vi "Poll DMA.vi"(8 "error in":errorcluster, 10 "Injection.Results":T13 {"Measurements"."Shots"."Results"."Off-Stage Min Volt" format="%#.6g"; "Measurements"."Shots"."Results"."Off-Stage Avg Volt" format="%#.6g"; "Measurements"."Shots"."Results"."Off-Stage Max Volt" format="%#.6g"; "Measurements"."Shots"."Results"."Total Stage Time (us)" format="%#.6g"; "Measurements"."Shots"."Results"."Off-Stage Avg Current" format="%#.6g"; "Measurements"."Shots"."Results"."Total Voltage Pulses" format="%#.6g"; "Measurements"."Shots"."Results"."Off-Stage Min Current" format="%#.6g"; "Measurements"."Shots"."Results"."Off-Stage Max Current" format="%#.6g"}, 11 "Parameters":T1) -> (0 "error out":errorcluster, 1 "Elements Remaining":u32, 3 "Parameters":T1)   [LabVIEW 2019, in "Fuel Injector Analysis Addon Engine.lvlib"]
uses:
  Fuel Injector Analysis Addon Engine.lvlib
  Types/Injector Event Data Cluster.ctl
  Types/Shot Information Control.ctl
  Types/Stage.Measurements.ctl
  Types/Async Parameters.ctl
  Addon Shared/Types/Shot.Parameters.ctl
  Addon Shared/Types/Stage.Parameters.ctl
  Addon Shared/Types/Stage.PullIn.Types.ctl
  Addon Shared/Types/Stage.Transition.Types.ctl
  Addon Shared/Types/Analysis.Channels.Select.ctl
  Addon Shared/Types/Injector info.ctl
  Types/Injector.State.ctl
  <vilib>/NI/NIVS Inline Async API/_Data Access Engine/Data Access Engine/Types/Write.DVR.ctl
  <vilib>/NI/NIVS Inline Async API/_Data Access Engine/Access Type Classes/Write/Write.lvclass
  <vilib>/NI/NIVS Inline Async API/_Data Access Engine/Data Access Engine/Types/Read.DVR.ctl
  <vilib>/NI/NIVS Inline Async API/_Data Access Engine/Access Type Classes/Read/Read.lvclass
  Addon Shared/Types/Compiled.Group.WaveformRefs.ctl
  <vilib>/NI VeriStand/Custom Device API/Waveform Data Reference.ctl
  <vilib>/NI VeriStand/Custom Device Waveform API/Single Waveform Write (DBL)/Single Waveform Write (DBL).lvclass
  C:/Program Files (x86)/National Instruments/LabVIEW 2019/vi.lib/NI VeriStand/Custom Device Waveform API/Waveform Session.lvclass
  <vilib>/NI/NIVS Inline Async API/_Data Access Engine/Access Type Classes/Read/Read.lvclass/Read.ctl
  <vilib>/NI VeriStand/Custom Device Waveform API/Waveform Session.lvclass/Waveform Session.ctl
  <vilib>/NI VeriStand/Custom Device Waveform API/Single Waveform Write (DBL)/Single Waveform Write (DBL).lvclass/Single Waveform Write (DBL).ctl
  <vilib>/NI VeriStand/Custom Device Waveform API/Internal Comm Classes/WPL Comm/WPL Comm (1D DBL)/WPL Comm (1D DBL).lvclass/WPL Comm (1D DBL).ctl
  <vilib>/NI VeriStand/Custom Device Waveform API/Internal Comm Classes/WPL Comm/WPL Comm.lvclass/WPL Comm.ctl
  <vilib>/NI/NIVS Inline Async API/_Data Access Engine/Access Type Classes/Write/Write.lvclass/Write.ctl
  Waveform Write.vi
  Stages.GetValues.vi
  Pack Data and Write to Inline.vi
  Build Event from Shots.vi
  Parse Injection Data.vi
  <vilib>/NI VeriStand/Custom Device Waveform API/NI VeriStand - Write Waveform(s).vi
  <vilib>/NI VeriStand/Custom Device Waveform API/Single Waveform Write (DBL)/NI VeriStand - Write Single Waveform (DBL).vi
  <vilib>/NI/NIVS Inline Async API/_Data Access Engine/Data Access Engine/Methods/Data.Processes.Execute.vi
  <vilib>/NI/NIVS Inline Async API/_Data Access Engine/Data Access Engine/Methods/Read.Data.vi
  Build Result Array from Shots.vi
  <vilib>/NI/NIVS Inline Async API/_Data Access Engine/Data Access Engine/Methods/Write.Data.vi
  Calculate Current Magnitude Measurements.vi
  RT.Stages.Find.vi
  <vilib>/NI VeriStand/Custom Device Waveform API/Internal Comm Classes/WPL Comm/WPL Comm (1D DBL)/Comm_write 1d dbl.vi
  <vilib>/NI VeriStand/Custom Device Waveform API/Read Sample offset DVR.vi
  <vilib>/NI VeriStand/Custom Device Waveform API/Check Opened.vi
  <vilib>/NI/NIVS Inline Async API/_Data Access Engine/Access Type Classes/Read/Read.ProcessData.vi
  <vilib>/NI/NIVS Inline Async API/_Data Access Engine/Access Type Classes/Write/Write.ProcessData.vi
  Calculate Hold-In Measurements.vi
  <vilib>/Analysis/baseanly.llb/Mean.vi
  <vilib>/Analysis/baseanly.llb/Mean (DBL).vi
  Calculate Voltage Pulses.vi
  Calculate Hold-In Voltage Measurements.vi
  <vilib>/NI VeriStand/Custom Device Waveform API/Internal Comm Classes/WPL Comm/Direct Send WPL Command.vi
  <vilib>/NI VeriStand/Custom Device Waveform API/Internal Comm Classes/WPL Comm/Convert Q Error to Shutdown Error.vi
  <vilib>/NI/NIVS Inline Async API/_Data Access Engine/Access Type Classes/Write/Write.Buffer.vi
  <vilib>/NI/NIVS Inline Async API/_Data Access Engine/Access Type Classes/Write/Write.Commit.vi
  <vilib>/NI VeriStand/Custom Device Waveform API/Internal Comm Classes/WPL Comm/WPL Comm (1D DBL)/WPL Comm (1D DBL).lvclass
  C:/Program Files (x86)/National Instruments/LabVIEW 2019/vi.lib/NI VeriStand/Custom Device Waveform API/Internal Comm Classes/WPL Comm/WPL Comm.lvclass
  <vilib>/Utility/error.llb/Error Cluster From Error Code.vi
  <vilib>/rvi/errors/niLvFpgaAdjustHostInterfaceError.vi
  Addon Shared/SubVIs/Constants.vi
  <vilib>/rvi/interface/nirviMethod/nirviMethod.xnode
  <vilib>/FPGAPlugInAG/Dynamic/niLvFpga_ReadFifo_Dynamic.vi
  <vilib>/rvi/errors/niLvFpgaMergeErrorWithErrorCode.vi
  Addon Shared/Fuel Injector Analysis Addon Shared.lvlib
  <vilib>/NI VeriStand/Custom Device API/Custom Device API.lvlib
  <vilib>/NI/NIVS Inline Async API/_Data Access Engine/Data Access Engine/Data Access Engine.lvclass
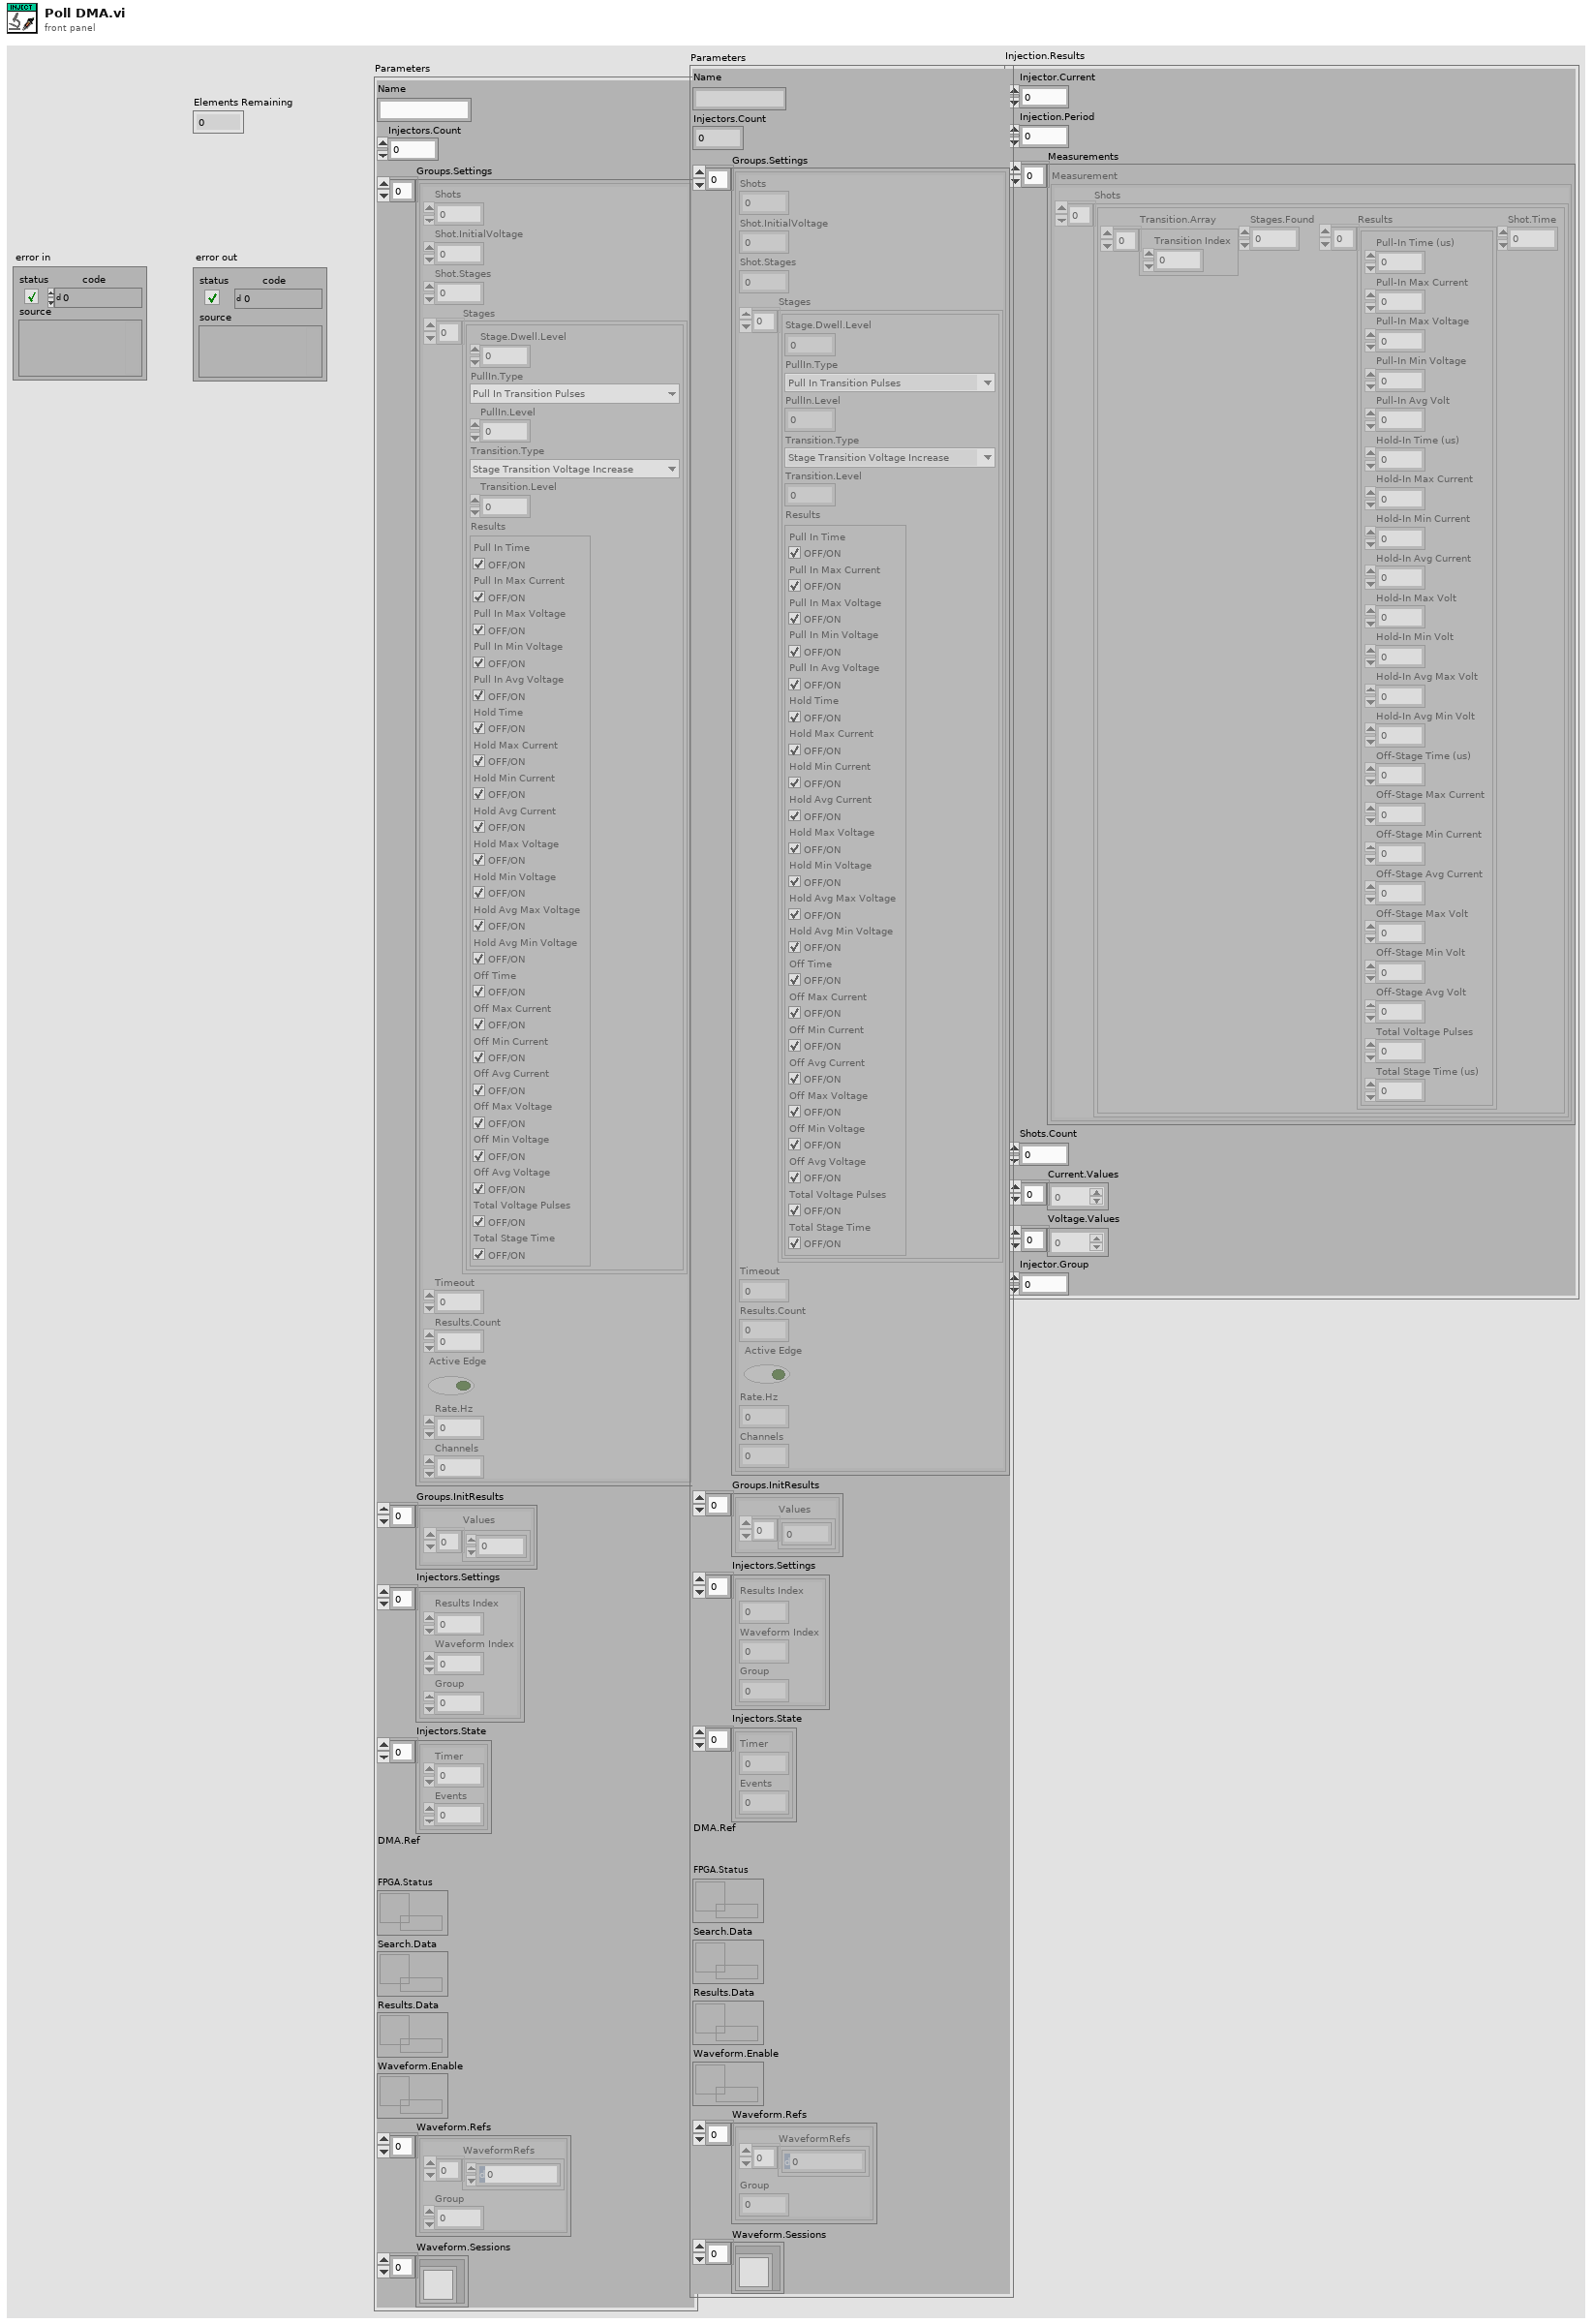
[diagram p1: front panel]
types:
  T1 = typedef "Fuel Injector Analysis Addon Engine.lvlib/Async Parameters.ctl" = cluster{"Name":string, "Injectors.Count":u8, "Groups.Settings":T2[], "Groups.InitResults":cluster{"Values":dbl[]}[], "Injectors.Settings":T7[], "Injectors.State":T8[], "DMA.Ref":refnum<k20>, "FPGA.Status":T9, "Search.Data":T10, "Results.Data":T9, "Waveform.Enable":T10, "Waveform.Refs":T11[], "Waveform.Sessions":refnum<class "Single Waveform Write (DBL).lvclass">[]}
  T2 = typedef "Fuel Injector Analysis Addon Shared.lvlib/Shot.Parameters.ctl" = cluster{"Shots":u32, "Shot.InitialVoltage":dbl, "Shot.Stages":u32, "Stages":T3[], "Timeout":dbl, "Results.Count":i32, "Active Edge":bool, "Rate.Hz":u32, "Channels":u32}
  T3 = typedef "Fuel Injector Analysis Addon Shared.lvlib/Stage.Parameters.ctl" = cluster{"Stage.Dwell.Level":dbl, "PullIn.Type":T4, "PullIn.Level":dbl, "Transition.Type":T5, "Transition.Level":dbl, "Results":T6}
  T4 = typedef "Fuel Injector Analysis Addon Shared.lvlib/Stage.PullIn.Types.ctl" = enum8{"Pull In Transition Pulses", "Pull In Transition Current Drop"}
  T5 = typedef "Fuel Injector Analysis Addon Shared.lvlib/Stage.Transition.Types.ctl" = enum8{"Stage Transition Inactive Time", "Stage Transition Voltage Increase", "Stage Transition Current Decrease", "Stage Transition Active Time"}
  T6 = typedef "Fuel Injector Analysis Addon Shared.lvlib/Analysis.Channels.Select.ctl" = cluster{"Pull In Time":bool, "Pull In Max Current":bool, "Pull In Max Voltage":bool, "Pull In Min Voltage":bool, "Pull In Avg Voltage":bool, "Hold Time":bool, "Hold Max Current":bool, "Hold Min Current":bool, "Hold Avg Current":bool, "Hold Max Voltage":bool, "Hold Min Voltage":bool, "Hold Avg Max Voltage":bool, "Hold Avg Min Voltage":bool, "Off Time":bool, "Off Max Current":bool, "Off Min Current":bool, "Off Avg Current":bool, "Off Max Voltage":bool, "Off Min Voltage":bool, "Off Avg Voltage":bool, "Total Voltage Pulses":bool, "Total Stage Time":bool}
  T7 = typedef "Fuel Injector Analysis Addon Shared.lvlib/Injector info.ctl" = cluster{"Results Index":i32, "Waveform Index":i32, "Group":u16}
  T8 = typedef "Fuel Injector Analysis Addon Engine.lvlib/Injector.State.ctl" = cluster{"Timer":u32, "Events":u64}
  T9 = typedef "Data Access Engine.lvlib/Data Access Engine.lvclass/Write.DVR.ctl" = refnum<data-value>
  T10 = typedef "Data Access Engine.lvlib/Data Access Engine.lvclass/Read.DVR.ctl" = refnum<data-value>
  T11 = typedef "Fuel Injector Analysis Addon Shared.lvlib/Compiled.Group.WaveformRefs.ctl" = cluster{"WaveformRefs":T12[], "Group":i32}
  T12 = typedef "Custom Device API.lvlib/Waveform Data Reference.ctl" = i32
  T13 = typedef "Fuel Injector Analysis Addon Engine.lvlib/Injector Event Data Cluster.ctl" = cluster{"Injector.Current":i16, "Injection.Period":dbl, "Measurements":cluster{"Shots":T14[]}[], "Shots.Count":i32, "Current.Values":dbl[], "Voltage.Values":dbl[], "Injector.Group":i16}
  T14 = typedef "Fuel Injector Analysis Addon Engine.lvlib/Shot Information Control.ctl" = cluster{"Transition.Array":i32[], "Stages.Found":u16, "Results":T15[], "Shot.Time":dbl}
  T15 = typedef "Fuel Injector Analysis Addon Engine.lvlib/Stage.Measurements.ctl" = cluster{"Pull-In Time (us)":dbl, "Pull-In Max Current":dbl, "Pull-In Max Voltage":dbl, "Pull-In Min Voltage":dbl, "Pull-In Avg Volt":dbl, "Hold-In Time (us)":dbl, "Hold-In Max Current":dbl, "Hold-In Min Current":dbl, "Hold-In Avg Current":dbl, "Hold-In Max Volt":dbl, "Hold-In Min Volt":dbl, "Hold-In Avg Max Volt":dbl, "Hold-In Avg Min Volt":dbl, "Off-Stage Time (us)":dbl, "Off-Stage Max Current":dbl, "Off-Stage Min Current":dbl, "Off-Stage Avg Current":dbl, "Off-Stage Max Volt":dbl, "Off-Stage Min Volt":dbl, "Off-Stage Avg Volt":dbl, "Total Voltage Pulses":dbl, "Total Stage Time (us)":dbl}
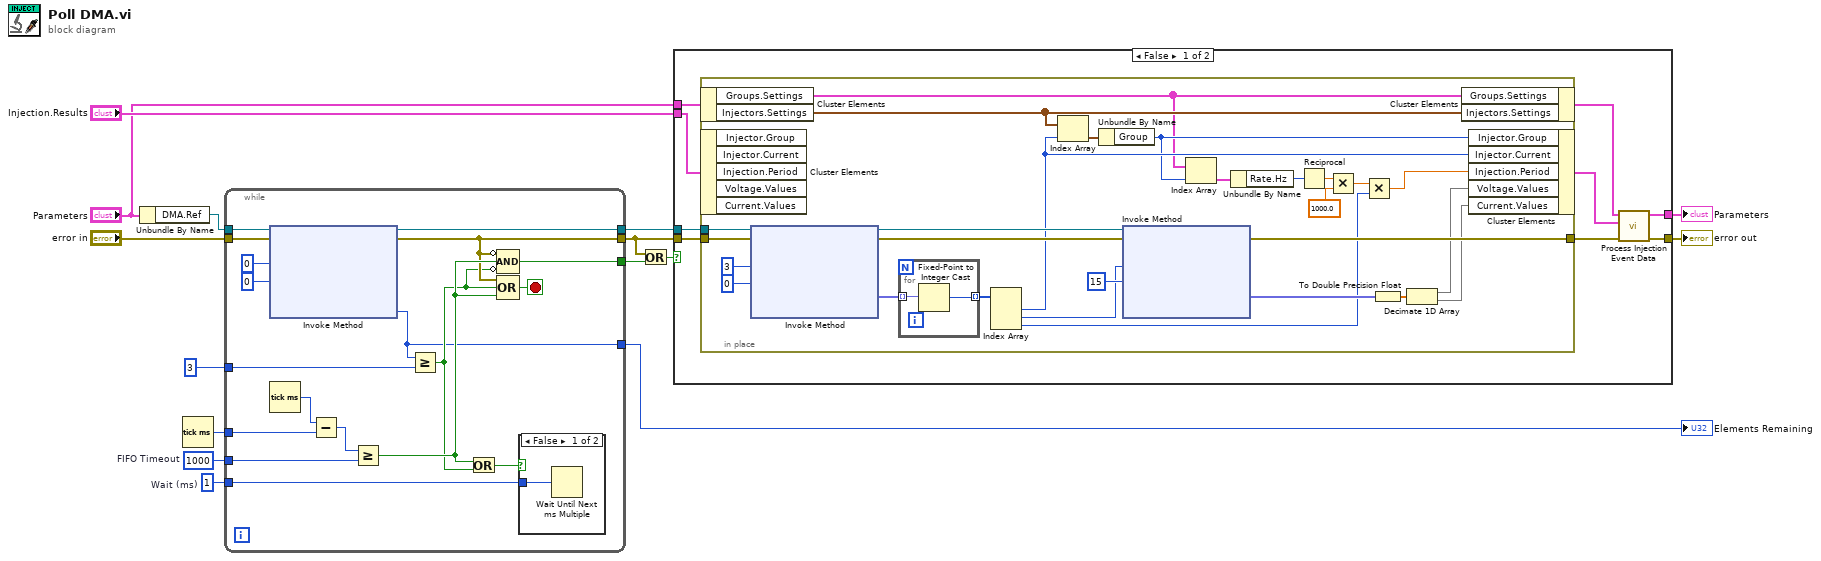
[diagram p0: block diagram]
diagram:
  w3 = u32 1  # Wait (ms)
  w4 = u32 1000  # FIFO Timeout
  n1 = Unbundle By Name("Parameters") -> ("DMA.Ref"=w7:refnum<k20>)
  n2 = Tick Count (ms)() -> (millisecond timer value=w14:u32)
  n3 = while {
    tunnel: "error in" -> [w33]
    tunnel: w3 -> [w32]
    tunnel: w14 -> [w29]
    tunnel: w4 -> [w27]
    tunnel: [w25] -> w10
    tunnel: [w20] -> w11
    tunnel: [w19] -> w12
    tunnel: w7 -> [w23]
    tunnel: u32 3 ("Number of Elements") -> [w17]
    tunnel: [w16] -> w1
    stop <- w24 stop-if-true
    n4 = xnode "Invoke Method"("FPGA VI Reference In"=w23, "error in"=w33, "Number of Elements"=u32 0, "Timeout (ms)"=0) -> ("FPGA VI Reference Out"=w25:refnum<k20>, "error out"=w20:errorcluster, "Elements Remaining"=w16:u32)  [unwired: 1 out]
    n5 = Tick Count (ms)() -> (millisecond timer value=w30:u32)
    n6 = Subtract(x=w30, y=w29) -> (x-y=w28:u32)
    n7 = Greater Or Equal?(x=w28, y=w27) -> (x >= y?=w21:bool)
    n8 = Greater Or Equal?(x=w16, y=w17) -> (x >= y?=w18:bool)
    n9 = Or(x=w21, y=w18) -> (x .or. y?=w26:bool)
    n10 = Compound Arithmetic op=AND(invert w20, w21, invert w18) -> (w19:bool)
    n11 = Compound Arithmetic op=OR(w20, w18, w21) -> (w24:bool)
    n12 = case shown="False" w26 {
      tunnel: w32 -> [w34 _]
      frame False {
        n13 = Wait Until Next ms Multiple(millisecond multiple=w34) -> ()  [unwired: 1 out]
      }
      frame True {
      }
    }
  }
  "Elements Remaining" <- w1
  n14 = Or(x=w11, y=w12) -> (x .or. y?=w13:bool)
  n15 = case shown="False" w13 {
    tunnel: w11 -> [w42 w74]
    tunnel: w10 -> [w43 _]
    tunnel: [w40 w74] -> w8
    tunnel: "Injection.Results" -> [w36 _]
    tunnel: "Parameters" -> [w38 w73]
    tunnel: [w39 w73] -> w5
    frame False {
      n16 = in-place {
        in-place-border: w43 -> [w70]
        in-place-border: w42 -> [w69]
        in-place-border: [w62] -> w41
        n17 = in-place-cluster #1(w38) -> ("Groups.Settings"=w46:T2[], "Injectors.Settings"=w48:T7[])
        n18 = in-place-cluster #2(w36) -> ()  [unwired: 5 out]
        n19 = xnode "Invoke Method"("FPGA VI Reference In"=w70, "error in"=w69, "Number of Elements"=u32 3, "Timeout (ms)"=0) -> ("FPGA VI Reference Out"=w65:refnum<k20>, "error out"=w64:errorcluster, "Data"=w67:fxp<+/-,32,8>[])  [unwired: 1 out]
        n20 = for {
          tunnel: w67 -> [w72] mode=indexing
          tunnel: [w71] -> w66 mode=indexing
          n21 = Fixed-Point to Integer Cast(1:w72) -> (0:w71:i32)
        }
        n22 = Index Array(array=w66) -> (element #1=w50:i32, element #2=w57:i32, element #3=w56:i32)  [unwired: 3 in]
        n23 = Index Array(array=w48, index=w50) -> (element=w49:T7)
        n24 = Unbundle By Name(w49) -> ("Group"=w47:u16)
        n25 = xnode "Invoke Method"("FPGA VI Reference In"=w65, "error in"=w64, "Number of Elements"=w57, "Timeout (ms)"=15) -> ("error out"=w62:errorcluster, "Data"=w61:fxp<+/-,32,8>[])  [unwired: 2 out]
        n26 = Index Array(array=w46, index=w47) -> (element=w45:T2)
        n27 = Unbundle By Name(w45) -> ("Rate.Hz"=w44:u32)
        n28 = Reciprocal(x=w44) -> (1/x=w59:dbl)
        n29 = Multiply(x=w59, y=1000.0) -> (x*y=w58:dbl)
        n30 = Multiply(x=w58, y=w56) -> (x*y=w54:dbl)
        n31 = To Double Precision Float(number=w61) -> (double precision float=w55:dbl[])
        n32 = Decimate 1D Array(w55) -> (w53:dbl[], w52:dbl[])
        n33 = in-place-cluster #1("Groups.Settings"=w46, "Injectors.Settings"=w48) -> (w37:T1)
        n34 = in-place-cluster #2("Injector.Group"=w47, "Injector.Current"=w50, "Injection.Period"=w54, "Voltage.Values"=w53, "Current.Values"=w52) -> (w35:T13)
      }
      n35 = call "Process Injection Event Data.vi"("error in (no error)"=w41, "Injection.Results"=w35, "Parameters"=w37) -> ("error out"=w40:errorcluster, "Parameters"=w39:T1)  [unwired: 7 in]
    }
    frame True {
    }
  }
  "error out" <- w8
  "Parameters" <- w5
